vi "event_interface_focus.vi"(6 "event_interface":refnum<user-event>, 8 "error in (no error)":errorcluster) -> (0 "error out":errorcluster)   [LabVIEW 2015, in "lv-interface-sub-re.lvlib"]
uses:
  lv-interface-sub-re.lvlib
  _controls/event_interface.ctl
  _controls/event_interface_command.ctl
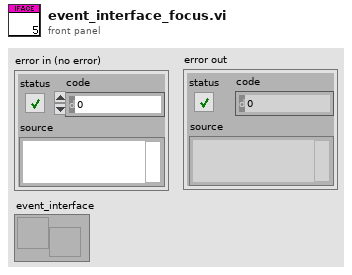
[diagram p1: front panel]
types:
  T1 = typedef "lv-interface-sub-re.lvlib/event_interface_command.ctl" = enum16{"<event_interface_cmd>", "defer_panel_updates", "focus", "unfocus", "undefer_panel_updates", "<null>"}
  T2 = typedef "lv-interface-sub-re.lvlib/event_interface.ctl" = cluster{"command":T1, "data":variant}
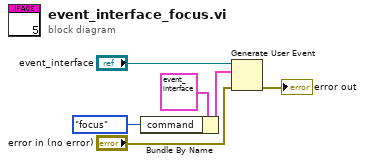
[diagram p0: block diagram]
diagram:
  n1 = Bundle By Name(cluster=T2 {"command"=enum."<event_interface_cmd>", "data"=variant} ("event data"), "command"=event_interface_command."focus") -> (w2:T2)
  n2 = Generate User Event(user event="event_interface", event data cluster=w2, error in="error in (no error)") -> (error out=→"error out":errorcluster)  [unwired: 1 in, 1 out]
